vi "Get SysDef Configuration.vi"(8 "error in (no error)":errorcluster, 11 "Node Ptr":T27 format="%.0x") -> (0 "error out":errorcluster, 3 "Configuration":T1={"Name"="", "Description"="", "Protocol"="", "RS232 Config"={"Port"="COM1", "Baud Rate"=9600, "Data Bits"=8, "Parity"=enum."None", "Stop Bits"=10, "Flow Control"=0, "XON"=enum."DC1", "XOFF"=enum."DC3", "End Read on Termination Character"=TRUE, "End Write on Termination Character"=TRUE, "Termination Character"=10}, "MetaData Globals"=[], "Message Groups"=[], "GPIB Config"={"VISA Resource"="GPIB0::2::INSTR", "Enable Termination Character"=TRUE, "Termination Character"=10, "Timeout"=2000, "Append Write Termination Character"=FALSE}, "TCPIP Config"={"IP Address"="localhost", "Port"=0}, "Decimation"=0, "UDP Config"={"Local IP Address"="localhost", "Local Port"=8888, "Target IP Address"="localhost", "Target Port"=8888}} {"GPIB Config"."Termination Character" format="%.0x"; "RS232 Config"."Termination Character" format="%.0x"; "RS232 Config"."Flow Control" items=["None"=0, "XON/XOFF"=1, "RTS/CTS"=2, "DTR/DSR"=4]; "RS232 Config"."Stop Bits" items=["1.0"=10, "1.5"=15, "2.0"=20]; "RS232 Config"."Data Bits" min=5 max=8 step=1; "RS232 Config"."Baud Rate" items=["75"=75, "110"=110, "134"=134, "150"=150, "300"=300, "600"=600, "1200"=1200, "1800"=1800, "2400"=2400, "4800"=4800, "7200"=7200, "9600"=9600, "14400"=14400, "19200"=19200, "28800"=28800, "38400"=38400, "56000"=56000, "57600"=57600, "115200"=115200, "128000"=128000, "230400"=230400, "460800"=460800, "921600"=921600, "1843200"=1843200, "3000000"=3000000]})   [LabVIEW 2019, in "Instrument Addon System Explorer.lvlib"]
uses:
  Instrument Addon System Explorer.lvlib
  <vilib>/NI VeriStand/Custom Device API/Custom Device Item Ref.ctl
  Instrument Custom Device SysDef Configuration V1.0.1.ctl
  Shared/Types/RSXXX Port Settings.ctl
  MetaData Channel Configuration.ctl
  Shared/Types/MetaData Parameters.ctl
  Shared/Types/Protocol Data Type.ctl
  Shared/Types/Metadata Channel Type.ctl
  Shared/Types/Type Cast Type.ctl
  Shared/Types/Endian.ctl
  Types/Channel Properties.ctl
  Message Group Configuration.ctl
  Message Configuration.ctl
  Command Message Configuration.ctl
  Shared/Types/Command Parameters.ctl
  Shared/Types/Linked Channel Cluster.ctl
  Response Message Configuration.ctl
  Shared/Types/Response Parameters.ctl
  Shared/Types/Response Wait Type.ctl
  Data Channel Configuration.ctl
  Shared/Types/Data Parameters.ctl
  Shared/Types/Data Channel Type.ctl
  Shared/Types/Message Parameters.ctl
  Shared/Types/Message Generation Type.ctl
  Shared/Types/Trigger Parameters.ctl
  Shared/Types/VISA Settings.ctl
  Shared/Types/TCPIP Settings.ctl
  Shared/Types/UDP Settings.ctl
  Shared/Types/FG Control.ctl
  Shared/Constants.vi
  <vilib>/NI VeriStand/Custom Device API/Get Item Property (U32).vi
  <vilib>/NI VeriStand/Custom Device API/NI VeriStand - Set Item Property.vi
  <vilib>/NI VeriStand/Custom Device API/Set Item Property (U32).vi
  <vilib>/NI VeriStand/Custom Device API/Get Item Property (String).vi
  <vilib>/NI VeriStand/Custom Device API/Set Item Property (String).vi
  <vilib>/NI VeriStand/Custom Device API/Get Item Property (Boolean).vi
  <vilib>/NI VeriStand/Custom Device API/Set Item Property (Boolean).vi
  <vilib>/NI VeriStand/Custom Device Tools/Custom Device Utility Library/NI VeriStand - Search for Item by GUID.vi
  <vilib>/NI VeriStand/Custom Device API/Get Item Property (String Array).vi
  <vilib>/NI VeriStand/Custom Device API/Set Item Property (String Array).vi
  <vilib>/NI VeriStand/Custom Device API/NI VeriStand - Set Custom Device Channel Value Table.vi
  <vilib>/NI VeriStand/Custom Device Tools/Custom Device Utility Library/NI VeriStand - Search for All Items by GUID.vi
  <vilib>/NI VeriStand/Custom Device API/Get Item Property (Double).vi
  <vilib>/NI VeriStand/Custom Device API/Set Item Property (Double).vi
  <vilib>/NI VeriStand/Custom Device API/Custom Device API.lvlib
  Shared/Instrument Addon Shared.lvlib
  <vilib>/NI VeriStand/Custom Device Tools/Custom Device Utility Library/Custom Device Utility Library.lvlib
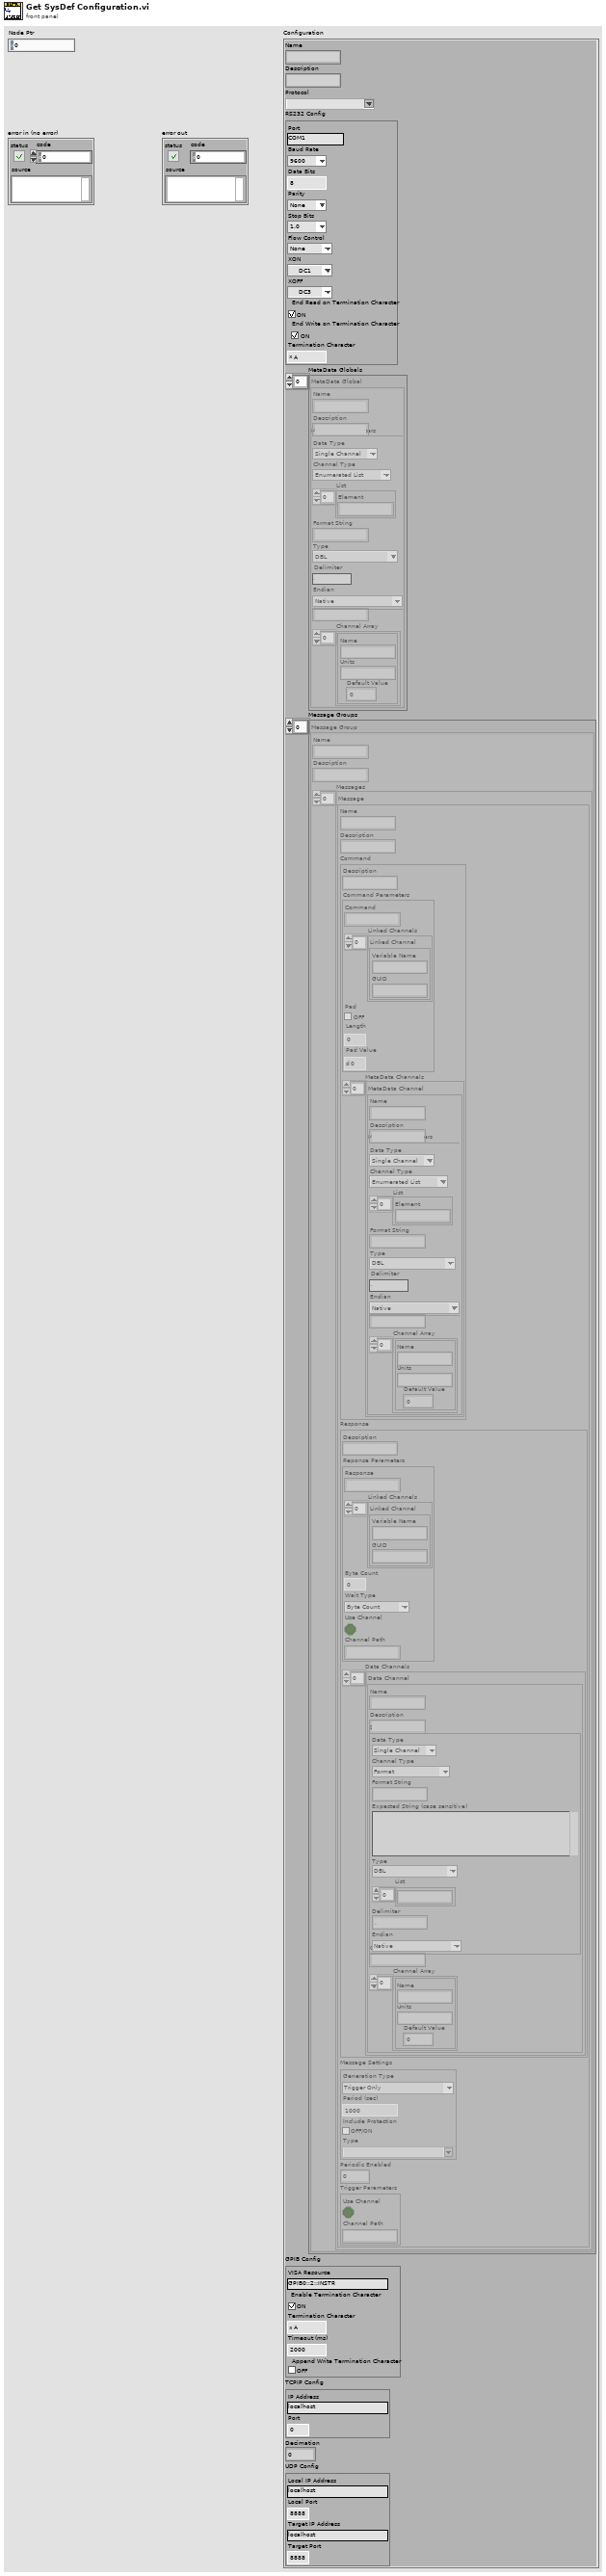
[diagram p1: front panel]
types:
  T1 = typedef "Instrument Addon System Explorer.lvlib/Instrument Custom Device SysDef Configuration V1.0.1.ctl" = cluster{"Name":string, "Description":string, "Protocol":string, "RS232 Config":T2, "MetaData Globals":T3[], "Message Groups":T10[], "GPIB Config":T24, "TCPIP Config":T25, "Decimation":u32, "UDP Config":T26}
  T2 = typedef "Instrument Addon Shared.lvlib/RSXXX Port Settings.ctl" = cluster{"Port":string, "Baud Rate":u32, "Data Bits":u16, "Parity":enum16{"None", "Odd", "Even", "Mark", "Space"}, "Stop Bits":u16, "Flow Control":u16, "XON":enum16{"NUL", "SOH", "STX", "ETX", "EOT", "ENQ", "ACK", "BEL", "BS", "HT", "LF", "VT", "FF", "CR", "SO", "SI", "DLE", "DC1", "DC2", "DC3", "DC4", "NAK", "SYN", "ETB", "CAN", "EM", "SUB", "ESC", "FS", "GS", "RS", "US", "SP", "!", "\"", "#", "$", "%", "&", "'", "(", ")", "*", "+", ",", "- (-)", ".", "/", "0", "1", "2", "3", "4", "5", "6", "7", "8", "9", ":", ";", "<", "=", ">", "?", "@", "A", "B", "C", "D", "E", "F", "G", "H", "I", "J", "K", "L", "M", "N", "O", "P", "Q", "R", "S", "T", "U", "V", "W", "X", "Y", "Z", "[", "\\", "]", "^", "_", "`", "a", "b", "c", "d", "e", "f", "g", "h", "i", "j", "k", "l", "m", "n", "o", "p", "q", "r", "s", "t", "u", "v", "w", "x", "y", "z", "{", "|", "}", "~"}, "XOFF":enum16{"NUL", "SOH", "STX", "ETX", "EOT", "ENQ", "ACK", "BEL", "BS", "HT", "LF", "VT", "FF", "CR", "SO", "SI", "DLE", "DC1", "DC2", "DC3", "DC4", "NAK", "SYN", "ETB", "CAN", "EM", "SUB", "ESC", "FS", "GS", "RS", "US", "SP", "!", "\"", "#", "$", "%", "&", "'", "(", ")", "*", "+", ",", "- (-)", ".", "/", "0", "1", "2", "3", "4", "5", "6", "7", "8", "9", ":", ";", "<", "=", ">", "?", "@", "A", "B", "C", "D", "E", "F", "G", "H", "I", "J", "K", "L", "M", "N", "O", "P", "Q", "R", "S", "T", "U", "V", "W", "X", "Y", "Z", "[", "\\", "]", "^", "_", "`", "a", "b", "c", "d", "e", "f", "g", "h", "i", "j", "k", "l", "m", "n", "o", "p", "q", "r", "s", "t", "u", "v", "w", "x", "y", "z", "{", "|", "}", "~"}, "End Read on Termination Character":bool, "End Write on Termination Character":bool, "Termination Character":u8}
  T3 = typedef "Instrument Addon System Explorer.lvlib/MetaData Channel Configuration.ctl" = cluster{"Name":string, "Description":string, "MetaData Parameters":T4, "Config GUID":string, "Channel Array":T9[]}
  T4 = typedef "Instrument Addon Shared.lvlib/MetaData Parameters.ctl" = cluster{"Data Type":T5, "Channel Type":T6, "List":string[], "Format String":string, "Type":T7, "Delimiter":string, "Endian":T8}
  T5 = typedef "Instrument Addon Shared.lvlib/Protocol Data Type.ctl" = enum16{"Single Channel", "Array"}
  T6 = typedef "Instrument Addon Shared.lvlib/Metadata Channel Type.ctl" = enum16{"Enumerated List", "Format", "Type Cast"}
  T7 = typedef "Instrument Addon Shared.lvlib/Type Cast Type.ctl" = enum16{"DBL", "SGL", "U64", "U32", "U16", "U8", "I64", "I32", "I16", "I8"}
  T8 = typedef "Instrument Addon Shared.lvlib/Endian.ctl" = enum16{"Native", "Little", "Big"}
  T9 = typedef "Instrument Addon System Explorer.lvlib/Channel Properties.ctl" = cluster{"Name":string, "Units":string, "Default Value":dbl}
  T10 = typedef "Instrument Addon System Explorer.lvlib/Message Group Configuration.ctl" = cluster{"Name":string, "Description":string, "Messages":T11[]}
  T11 = typedef "Instrument Addon System Explorer.lvlib/Message Configuration.ctl" = cluster{"Name":string, "Description":string, "Command":T12, "Response":T15, "Message Settings":T21, "Periodic Enabled":dbl, "Trigger Parameters":T23}
  T12 = typedef "Instrument Addon System Explorer.lvlib/Command Message Configuration.ctl" = cluster{"Description":string, "Command Parameters":T13, "MetaData Channels":T3[]}
  T13 = typedef "Instrument Addon Shared.lvlib/Command Parameters.ctl" = cluster{"Command":string, "Linked Channels":T14[], "Pad":bool, "Length":u32, "Pad Value":u8}
  T14 = typedef "Instrument Addon Shared.lvlib/Linked Channel Cluster.ctl" = cluster{"Variable Name":string, "GUID":string}
  T15 = typedef "Instrument Addon System Explorer.lvlib/Response Message Configuration.ctl" = cluster{"Description":string, "Reponse Parameters":T16, "Data Channels":T18[]}
  T16 = typedef "Instrument Addon Shared.lvlib/Response Parameters.ctl" = cluster{"Response":string, "Linked Channels":T14[], "Type Value":dbl, "Wait Type":T17, "Use Channel":bool, "Channel Path":string}
  T17 = typedef "Instrument Addon Shared.lvlib/Response Wait Type.ctl" = enum16{"Byte Count", "Wait sec"}
  T18 = typedef "Instrument Addon System Explorer.lvlib/Data Channel Configuration.ctl" = cluster{"Name":string, "Description":string, "Data Parameters":T19, "Config GUID":string, "Channel Array":T9[]}
  T19 = typedef "Instrument Addon Shared.lvlib/Data Parameters.ctl" = cluster{"Data Type":T5, "Channel Type":T20, "Format String":string, "Expected String":string, "Type":T7, "List":string[], "Delimiter":string, "Endian":T8}
  T20 = typedef "Instrument Addon Shared.lvlib/Data Channel Type.ctl" = enum16{"Format", "Comparison", "Type Cast", "Enumerated List"}
  T21 = typedef "Instrument Addon Shared.lvlib/Message Parameters.ctl" = cluster{"Generation Type":T22, "Period":dbl, "Include Protection":bool, "Type":string}
  T22 = typedef "Instrument Addon Shared.lvlib/Message Generation Type.ctl" = enum16{"Trigger Only", "Periodic & Trigger", "Value Change & Trigger"}
  T23 = typedef "Instrument Addon Shared.lvlib/Trigger Parameters.ctl" = cluster{"Use Channel":bool, "Channel Path":string}
  T24 = typedef "Instrument Addon Shared.lvlib/VISA Settings.ctl" = cluster{"VISA Resource":string, "Enable Termination Character":bool, "Termination Character":u8, "Timeout":u32, "Append Write Termination Character":bool}
  T25 = typedef "Instrument Addon Shared.lvlib/TCPIP Settings.ctl" = cluster{"IP Address":string, "Port":u16}
  T26 = typedef "Instrument Addon Shared.lvlib/UDP Settings.ctl" = cluster{"Local IP Address":string, "Local Port":u16, "Target IP Address":string, "Target Port":u16}
  T27 = typedef "Custom Device API.lvlib/Custom Device Item Ref.ctl" = u64
  T28 = typedef "Instrument Addon Shared.lvlib/FG Control.ctl" = enum16{"Get", "Set"}
  T29 = typedef "Custom Device API.lvlib/Custom Device Item Info.ctl" = cluster{"Name":string, "Is Channel":bool, "GUID":string, "Is Waveform":bool}
  T30 = typedef "Custom Device API.lvlib/Custom Device Channel.ctl" = cluster{"Type":T31, "Units":string, "Default Value":dbl, "Faultable":bool, "Scalable":bool}
  T31 = typedef "Custom Device API.lvlib/Custom Device Channel Type.ctl" = enum16{"Input", "Output"}
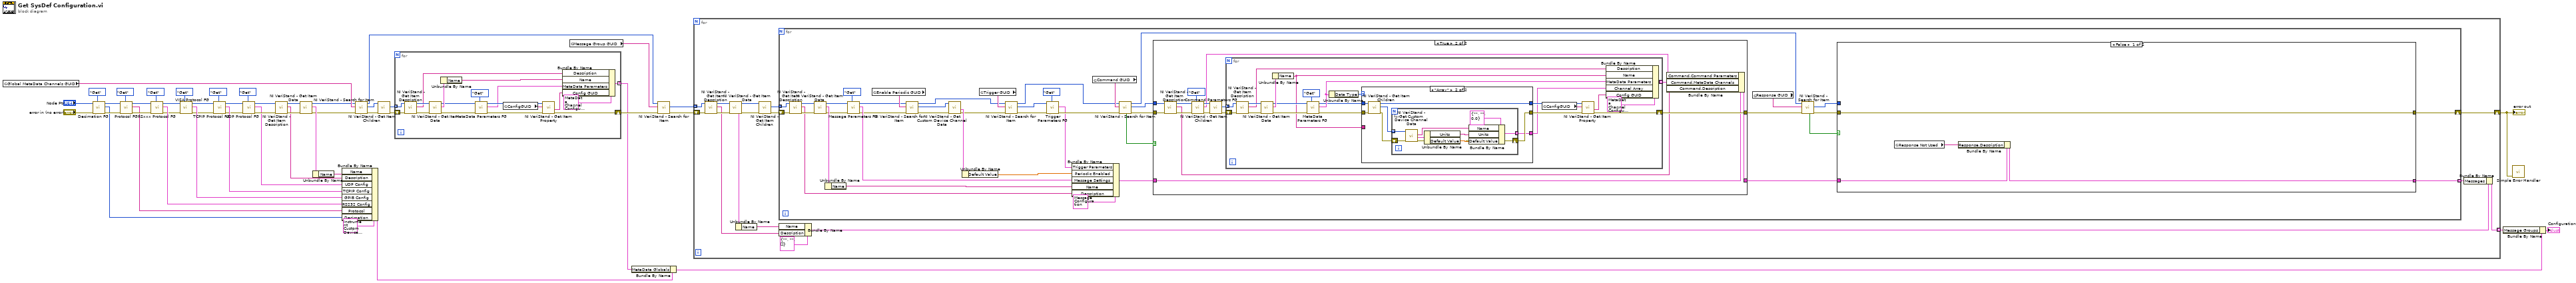
[diagram p0: block diagram]
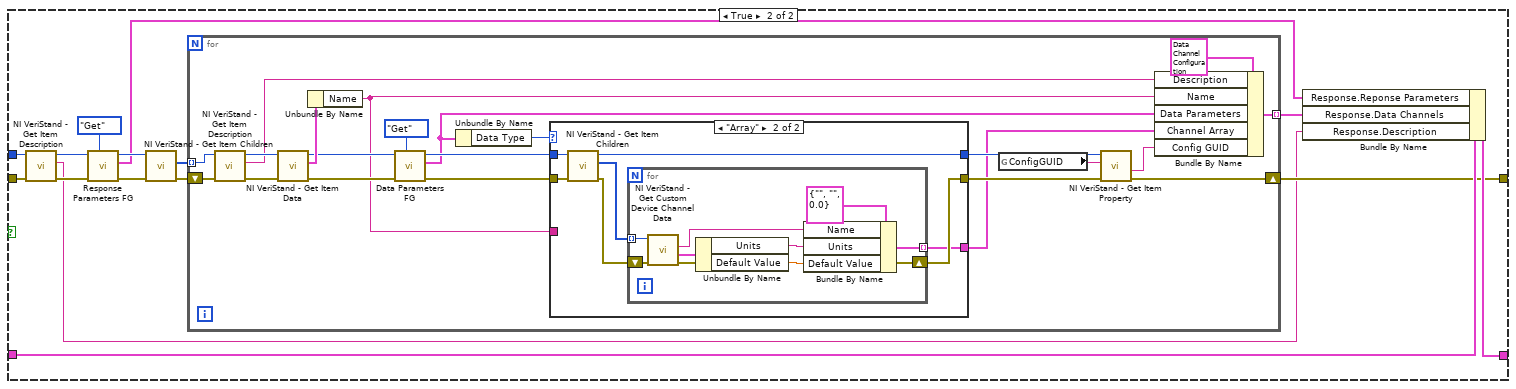
[diagram p2: hidden frame]
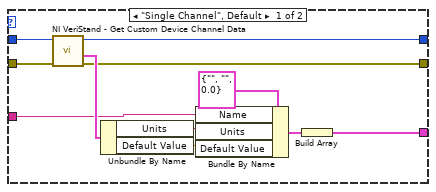
[diagram p3: hidden frame]
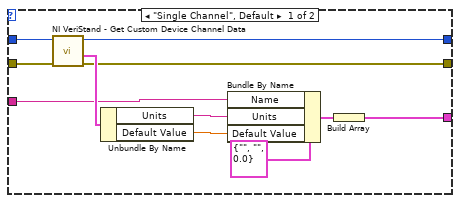
[diagram p5: hidden frame]
diagram:
  n1 = global read "Constants.vi" "Global MetaData Channels GUID"() -> (w46:string)
  n2 = call "Decimation FG.vi"("Action"=FG_Control."Get", "error in (no error)"="error in (no error)", "Device Item Ref in"="Node Ptr") -> ("error out"=w10:errorcluster, "Decimation out"=w7:u32, "Item Ref out"=w8:T27)  [unwired: 6 in]
  n3 = call "Protocol FG.vi"("Action"=FG_Control."Get", "error in (no error)"=w10, "Device Item Ref in"=w8) -> ("error out"=w43:errorcluster, "Protocol out"=w27:string, "Item Ref out"=w48:T27)  [unwired: 6 in]
  n4 = call "RSxxx Protocol FG.vi"("Action"=FG_Control."Get", "error in (no error)"=w43, "Device Item Ref in"=w48) -> ("error out"=w21:errorcluster, "Serial Config"=w25:T2, "Item Ref out"=w20:T27)  [unwired: 6 in]
  n5 = call "VISA Protocol FG.vi"("Action"=FG_Control."Get", "error in (no error)"=w21, "Device Item Ref in"=w20) -> ("error out"=w16:errorcluster, "VISA Config"=w19:T24, "Item Ref out"=w15:T27)  [unwired: 6 in]
  n6 = call "TCPIP Protocol FG.vi"("Action"=FG_Control."Get", "error in (no error)"=w16, "Device Item Ref in"=w15) -> ("error out"=w6:errorcluster, "TCP/IP Config"=w13:T25, "Item Ref out"=w4:T27)  [unwired: 6 in]
  n7 = call "UDP Protocol FG.vi"("Action"=FG_Control."Get", "error in (no error)"=w6, "Device Item Ref in"=w4) -> ("error out"=w5:errorcluster, "UDP Config"=w1:T26, "Item Ref out"=w3:T27)  [unwired: 6 in]
  n8 = call <vilib>:"NI VeriStand - Get Item Description.vi"("error in (no error)"=w5, "Item Ref in"=w3) -> ("error out"=w44:errorcluster, "Description"=w26:string, "Item Ref out"=w42:T27)  [unwired: 7 out]
  n9 = call <vilib>:"NI VeriStand - Get Item Data.vi"("error in (no error)"=w44, "Item Ref in"=w42) -> ("error out"=w40:errorcluster, "Item Info"=w50:T29, "Item Ref out"=w41:T27)  [unwired: 7 out]
  n10 = Unbundle By Name(w50) -> ("Name"=w24:string)
  n11 = Bundle By Name(cluster=T1 {"Name"="", "Description"="", "Protocol"="", "RS232 Config"={"Port"="", "Baud Rate"=0, "Data Bits"=0, "Parity"=enum."None", "Stop Bits"=0, "Flow Control"=0, "XON"=enum."NUL", "XOFF"=enum."NUL", "End Read on Termination Character"=FALSE, "End Write on Termination Character"=FALSE, "Termination Character"=0}, "MetaData Globals"=[], "Message Groups"=[], "GPIB Config"={"VISA Resource"="", "Enable Termination Character"=FALSE, "Termination Character"=0, "Timeout"=0, "Append Write Termination Character"=FALSE}, "TCPIP Config"={"IP Address"="", "Port"=0}, "Decimation"=0, "UDP Config"={"Local IP Address"="", "Local Port"=0, "Target IP Address"="", "Target Port"=0}}, "Name"=w24, "Description"=w26, "UDP Config"=w1, "TCPIP Config"=w13, "GPIB Config"=w19, "RS232 Config"=w25, "Protocol"=w27, "Decimation"=w7) -> (w22:T1)
  n12 = call-poly <vilib>:"NI VeriStand - Search for Item.vi"("error in"=w40, "Item GUID"=w46, "Section Ref in"=w41) -> ("error out"=w38:errorcluster, "Item Ref"=w45:T27, "Section Ref out"=w34:T27)  [unwired: 5 in, 1 out]
  n13 = call <vilib>:"NI VeriStand - Get Item Children.vi"("error in (no error)"=w38, "Item Ref in"=w45) -> ("error out"=w37:errorcluster, "Child Refs"=w39:T27[])  [unwired: 6 in, 2 out]
  n14 = for {
    tunnel: w39 -> [w65] mode=indexing
    shift-right: [w57] -> w35
    shift-left: w37 -> [w64]
    tunnel: [w51] -> w31 mode=indexing
    n15 = call <vilib>:"NI VeriStand - Get Item Description.vi"("error in (no error)"=w64, "Item Ref in"=w65) -> ("error out"=w67:errorcluster, "Description"=w52:string, "Item Ref out"=w68:T27)  [unwired: 7 out]
    n16 = call <vilib>:"NI VeriStand - Get Item Data.vi"("error in (no error)"=w67, "Item Ref in"=w68) -> ("error out"=w59:errorcluster, "Item Info"=w66:T29, "Item Ref out"=w58:T27)  [unwired: 7 out]
    n17 = Unbundle By Name(w66) -> ("Name"=w53:string)
    n18 = call "MetaData Parameters FG.vi"("Action"=FG_Control."Get", "error in (no error)"=w59, "Item Ref in"=w58) -> ("error out"=w61:errorcluster, "MetaData Parameters"=w54:T4, "Item Ref out"=w60:T27)  [unwired: 6 in]
    n19 = global read "Constants.vi" "ConfigGUID"() -> (w62:string)
    n20 = call-poly <vilib>:"NI VeriStand - Get Item Property.vi"("error in (no error)"=w61, "Property Name"=w62, "Item Ref in"=w60) -> ("error out"=w57:errorcluster, "Value"=w55:string)  [unwired: 5 in, 2 out]
    n21 = Bundle By Name(cluster=T3 {"Name"="", "Description"="", "MetaData Parameters"={"Data Type"=enum."Single Channel", "Channel Type"=enum."Enumerated List", "List"=[], "Format String"="", "Type"=enum."DBL", "Delimiter"="", "Endian"=enum."Native"}, "Config GUID"="", "Channel Array"=[]}, "Description"=w52, "Name"=w53, "MetaData Parameters"=w54, "Config GUID"=w55) -> (w51:T3)
  }
  n22 = global read "Constants.vi" "Message Group GUID"() -> (w36:string)
  n23 = Bundle By Name(cluster=w22, "MetaData Globals"=w31) -> (w30:T1)
  n24 = call-poly <vilib>:"NI VeriStand - Search for Item.vi"("error in"=w35, "Item GUID"=w36, "Section Ref in"=w34) -> ("error out"=w33:errorcluster, "Item Refs"=w32:T27[])  [unwired: 5 in, 2 out]
  n25 = for {
    tunnel: w32 -> [w80] mode=indexing
    tunnel: [w70] -> w29 mode=indexing
    shift-right: [w69] -> w17
    shift-left: w33 -> [w81]
    n26 = call <vilib>:"NI VeriStand - Get Item Description.vi"("error in (no error)"=w81, "Item Ref in"=w80) -> ("error out"=w83:errorcluster, "Description"=w73:string, "Item Ref out"=w82:T27)  [unwired: 7 out]
    n27 = call <vilib>:"NI VeriStand - Get Item Data.vi"("error in (no error)"=w83, "Item Ref in"=w82) -> ("error out"=w78:errorcluster, "Item Info"=w84:T29, "Item Ref out"=w79:T27)  [unwired: 7 out]
    n28 = Unbundle By Name(w84) -> ("Name"=w74:string)
    n29 = call <vilib>:"NI VeriStand - Get Item Children.vi"("error in (no error)"=w78, "Item Ref in"=w79) -> ("error out"=w77:errorcluster, "Child Refs"=w76:T27[])  [unwired: 6 in, 2 out]
    n30 = for {
      tunnel: w76 -> [w121] mode=indexing
      tunnel: [w112] -> w72 mode=indexing
      shift-right: [w111] -> w69
      shift-left: w77 -> [w122]
      n31 = call <vilib>:"NI VeriStand - Get Item Description.vi"("error in (no error)"=w122, "Item Ref in"=w121) -> ("error out"=w124:errorcluster, "Description"=w115:string, "Item Ref out"=w125:T27)  [unwired: 7 out]
      n32 = call <vilib>:"NI VeriStand - Get Item Data.vi"("error in (no error)"=w124, "Item Ref in"=w125) -> ("error out"=w103:errorcluster, "Item Info"=w123:T29, "Item Ref out"=w102:T27)  [unwired: 7 out]
      n33 = Unbundle By Name(w123) -> ("Name"=w116:string)
      n34 = call "Message Parameters FG.vi"("Action"=FG_Control."Get", "error in (no error)"=w103, "Item Ref in"=w102) -> ("error out"=w99:errorcluster, "Message Settings out"=w100:T21, "Item Ref out"=w98:T27)  [unwired: 6 in]
      n35 = global read "Constants.vi" "Enable Periodic GUID"() -> (w104:string)
      n36 = call-poly <vilib>:"NI VeriStand - Search for Item.vi"("error in"=w99, "Item GUID"=w104, "Section Ref in"=w98) -> ("error out"=w97:errorcluster, "Item Ref"=w95:T27, "Section Ref out"=w91:T27)  [unwired: 5 in, 1 out]
      n37 = call <vilib>:"NI VeriStand - Get Custom Device Channel Data.vi"("error in (no error)"=w97, "Channel Ref in"=w95) -> ("error out"=w92:errorcluster, "Channel"=w94:T30)  [unwired: 4 in, 4 out]
      n38 = Unbundle By Name(w94) -> ("Default Value"=w96:dbl)
      n39 = global read "Constants.vi" "Trigger GUID"() -> (w93:string)
      n40 = call-poly <vilib>:"NI VeriStand - Search for Item.vi"("error in"=w92, "Item GUID"=w93, "Section Ref in"=w91) -> ("error out"=w90:errorcluster, "Item Ref"=w88:T27, "Section Ref out"=w87:T27)  [unwired: 5 in, 1 out]
      n41 = call "Trigger Parameters FG.vi"("Action"=FG_Control."Get", "error in (no error)"=w90, "Item Ref in"=w88) -> ("error out"=w89:errorcluster, "Trigger Parameters"=w86:T23)  [unwired: 6 in, 1 out]
      n42 = Bundle By Name(cluster=T11 {"Name"="", "Description"="", "Command"={"Description"="", "Command Parameters"={"Command"="", "Linked Channels"=[], "Pad"=FALSE, "Length"=0, "Pad Value"=0}, "MetaData Channels"=[]}, "Response"={"Description"="", "Reponse Parameters"={"Response"="", "Linked Channels"=[], "Type Value"=0.0, "Wait Type"=enum."Byte Count", "Use Channel"=FALSE, "Channel Path"=""}, "Data Channels"=[]}, "Message Settings"={"Generation Type"=enum."Trigger Only", "Period"=0.0, "Include Protection"=FALSE, "Type"=""}, "Periodic Enabled"=0.0, "Trigger Parameters"={"Use Channel"=FALSE, "Channel Path"=""}}, "Trigger Parameters"=w86, "Periodic Enabled"=w96, "Message Settings"=w100, "Name"=w116, "Description"=w115) -> (w114:T11)
      n43 = global read "Constants.vi" "Command GUID"() -> (w126:string)
      n44 = call-poly <vilib>:"NI VeriStand - Search for Item.vi"("error in"=w89, "Item GUID"=w126, "Section Ref in"=w87) -> ("error out"=w109:errorcluster, "Item Ref"=w110:T27, "Section Ref out"=w118:T27, "Found"=w106:bool)  [unwired: 5 in]
      n45 = case shown="True" w106 {
        tunnel: [w195 w206] -> w119
        tunnel: w114 -> [w196 w203]
        tunnel: [w196 w202] -> w113
        tunnel: w110 -> [_ w201]
        tunnel: w109 -> [w195 w200]
        frame False {
        }
        frame True {
          n46 = call <vilib>:"NI VeriStand - Get Item Description.vi"("error in (no error)"=w200, "Item Ref in"=w201) -> ("error out"=w199:errorcluster, "Description"=w197:string, "Item Ref out"=w198:T27)  [unwired: 7 out]
          n47 = call "Command Parameters FG.vi"("Action"=FG_Control."Get", "error in (no error)"=w199, "Item Ref in"=w198) -> ("error out"=w210:errorcluster, "Command Parameters"=w205:T13, "Item Ref out"=w207:T27)  [unwired: 6 in]
          n48 = call <vilib>:"NI VeriStand - Get Item Children.vi"("error in (no error)"=w210, "Item Ref in"=w207) -> ("error out"=w209:errorcluster, "Child Refs"=w208:T27[])  [unwired: 6 in, 2 out]
          n49 = for {
            tunnel: w208 -> [w230] mode=indexing
            shift-right: [w224] -> w206
            shift-left: w209 -> [w229]
            tunnel: [w220] -> w204 mode=indexing
            n50 = call <vilib>:"NI VeriStand - Get Item Description.vi"("error in (no error)"=w229, "Item Ref in"=w230) -> ("error out"=w232:errorcluster, "Description"=w221:string, "Item Ref out"=w233:T27)  [unwired: 7 out]
            n51 = call <vilib>:"NI VeriStand - Get Item Data.vi"("error in (no error)"=w232, "Item Ref in"=w233) -> ("error out"=w226:errorcluster, "Item Info"=w231:T29, "Item Ref out"=w225:T27)  [unwired: 7 out]
            n52 = Unbundle By Name(w231) -> ("Name"=w213:string)
            n53 = call "MetaData Parameters FG.vi"("Action"=FG_Control."Get", "error in (no error)"=w226, "Item Ref in"=w225) -> ("error out"=w215:errorcluster, "MetaData Parameters"=w219:T4, "Item Ref out"=w217:T27)  [unwired: 6 in]
            n54 = Unbundle By Name(w219) -> ("Data Type"=w218:T5)
            n55 = case shown="\"Array\"" w218 {
              tunnel: w217 -> [w241 w251]
              tunnel: [w240 w250] -> w216
              tunnel: w215 -> [w243 w249]
              tunnel: [w242 w246] -> w214
              tunnel: [w235 w245] -> w212
              tunnel: w213 -> [w237 _]
              frame "Single Channel", Default {
                n56 = call <vilib>:"NI VeriStand - Get Custom Device Channel Data.vi"("error in (no error)"=w243, "Channel Ref in"=w241) -> ("error out"=w242:errorcluster, "Channel"=w244:T30, "Channel Ref out"=w240:T27)  [unwired: 4 in, 3 out]
                n57 = Unbundle By Name(w244) -> ("Units"=w238:string, "Default Value"=w239:dbl)
                n58 = Bundle By Name(cluster=T9 {"Name"="", "Units"="", "Default Value"=0.0}, "Name"=w237, "Units"=w238, "Default Value"=w239) -> (w236:T9)
                n59 = Build Array(w236) -> (w235:T9[])
              }
              frame "Array" {
                n60 = call <vilib>:"NI VeriStand - Get Item Children.vi"("error in (no error)"=w249, "Item Ref in"=w251) -> ("error out"=w247:errorcluster, "Child Refs"=w248:T27[], "Item Ref out"=w250:T27)  [unwired: 6 in, 1 out]
                n61 = for {
                  tunnel: w248 -> [w260] mode=indexing
                  tunnel: [w255] -> w245 mode=indexing
                  shift-right: [w253] -> w246
                  shift-left: w247 -> [w254]
                  n62 = call <vilib>:"NI VeriStand - Get Custom Device Channel Data.vi"("error in (no error)"=w254, "Channel Ref in"=w260) -> ("error out"=w253:errorcluster, "Channel"=w259:T30, "Channel Name"=w258:string)  [unwired: 4 in, 3 out]
                  n63 = Unbundle By Name(w259) -> ("Units"=w257:string, "Default Value"=w256:dbl)
                  n64 = Bundle By Name(cluster=T9 {"Name"="", "Units"="", "Default Value"=0.0}, "Name"=w258, "Units"=w257, "Default Value"=w256) -> (w255:T9)
                }
              }
            }
            n65 = global read "Constants.vi" "ConfigGUID"() -> (w227:string)
            n66 = call-poly <vilib>:"NI VeriStand - Get Item Property.vi"("error in (no error)"=w214, "Property Name"=w227, "Item Ref in"=w216) -> ("error out"=w224:errorcluster, "Value"=w222:string)  [unwired: 5 in, 2 out]
            n67 = Bundle By Name(cluster=T3 {"Name"="", "Description"="", "MetaData Parameters"={"Data Type"=enum."Single Channel", "Channel Type"=enum."Enumerated List", "List"=[], "Format String"="", "Type"=enum."DBL", "Delimiter"="", "Endian"=enum."Native"}, "Config GUID"="", "Channel Array"=[]}, "Description"=w221, "Name"=w213, "MetaData Parameters"=w219, "Channel Array"=w212, "Config GUID"=w222) -> (w220:T3)
          }
          n68 = Bundle By Name(cluster=w203, "Command.Command Parameters"=w205, "Command.MetaData Channels"=w204, "Command.Description"=w197) -> (w202:T11)
        }
      }
      n69 = global read "Constants.vi" "Response GUID"() -> (w120:string)
      n70 = call-poly <vilib>:"NI VeriStand - Search for Item.vi"("error in"=w119, "Item GUID"=w120, "Section Ref in"=w118) -> ("error out"=w108:errorcluster, "Item Ref"=w107:T27, "Found"=w105:bool)  [unwired: 5 in, 1 out]
      n71 = case shown="False" w105 {
        tunnel: w113 -> [w129 w138]
        tunnel: [w128 w137] -> w112
        tunnel: [w130 w136] -> w111
        tunnel: w108 -> [w130 w135]
        tunnel: w107 -> [_ w133]
        frame False {
          n72 = global read "Constants.vi" "Response Not Used"() -> (w127:string)
          n73 = Bundle By Name(cluster=w129, "Response.Description"=w127) -> (w128:T11)
        }
        frame True {
          n74 = call <vilib>:"NI VeriStand - Get Item Description.vi"("error in (no error)"=w135, "Item Ref in"=w133) -> ("error out"=w134:errorcluster, "Description"=w131:string, "Item Ref out"=w132:T27)  [unwired: 7 out]
          n75 = call "Response Parameters FG.vi"("Action"=FG_Control."Get", "error in (no error)"=w134, "Item Ref in"=w132) -> ("error out"=w142:errorcluster, "Reponse Parameters"=w139:T16, "Item Ref out"=w141:T27)  [unwired: 6 in]
          n76 = call <vilib>:"NI VeriStand - Get Item Children.vi"("error in (no error)"=w142, "Item Ref in"=w141) -> ("error out"=w144:errorcluster, "Child Refs"=w145:T27[])  [unwired: 6 in, 2 out]
          n77 = for {
            tunnel: w145 -> [w164] mode=indexing
            shift-right: [w161] -> w136
            shift-left: w144 -> [w163]
            tunnel: [w154] -> w140 mode=indexing
            n78 = call <vilib>:"NI VeriStand - Get Item Description.vi"("error in (no error)"=w163, "Item Ref in"=w164) -> ("error out"=w166:errorcluster, "Description"=w156:string, "Item Ref out"=w167:T27)  [unwired: 7 out]
            n79 = call <vilib>:"NI VeriStand - Get Item Data.vi"("error in (no error)"=w166, "Item Ref in"=w167) -> ("error out"=w159:errorcluster, "Item Info"=w165:T29, "Item Ref out"=w158:T27)  [unwired: 7 out]
            n80 = Unbundle By Name(w165) -> ("Name"=w146:string)
            n81 = call "Data Parameters FG.vi"("Action"=FG_Control."Get", "error in (no error)"=w159, "Item Ref in"=w158) -> ("error out"=w153:errorcluster, "Data Parameters"=w149:T19, "Item Ref out"=w151:T27)  [unwired: 6 in]
            n82 = Unbundle By Name(w149) -> ("Data Type"=w148:T5)
            n83 = case shown="\"Array\"" w148 {
              tunnel: w151 -> [w175 w185]
              tunnel: [w174 w184] -> w150
              tunnel: w153 -> [w177 w183]
              tunnel: [w176 w180] -> w152
              tunnel: [w169 w179] -> w147
              tunnel: w146 -> [w171 _]
              frame "Single Channel", Default {
                n84 = call <vilib>:"NI VeriStand - Get Custom Device Channel Data.vi"("error in (no error)"=w177, "Channel Ref in"=w175) -> ("error out"=w176:errorcluster, "Channel"=w178:T30, "Channel Ref out"=w174:T27)  [unwired: 4 in, 3 out]
                n85 = Unbundle By Name(w178) -> ("Units"=w172:string, "Default Value"=w173:dbl)
                n86 = Bundle By Name(cluster=T9 {"Name"="", "Units"="", "Default Value"=0.0}, "Name"=w171, "Units"=w172, "Default Value"=w173) -> (w170:T9)
                n87 = Build Array(w170) -> (w169:T9[])
              }
              frame "Array" {
                n88 = call <vilib>:"NI VeriStand - Get Item Children.vi"("error in (no error)"=w183, "Item Ref in"=w185) -> ("error out"=w181:errorcluster, "Child Refs"=w182:T27[], "Item Ref out"=w184:T27)  [unwired: 6 in, 1 out]
                n89 = for {
                  tunnel: w182 -> [w194] mode=indexing
                  tunnel: [w189] -> w179 mode=indexing
                  shift-right: [w187] -> w180
                  shift-left: w181 -> [w188]
                  n90 = call <vilib>:"NI VeriStand - Get Custom Device Channel Data.vi"("error in (no error)"=w188, "Channel Ref in"=w194) -> ("error out"=w187:errorcluster, "Channel"=w193:T30, "Channel Name"=w192:string)  [unwired: 4 in, 3 out]
                  n91 = Unbundle By Name(w193) -> ("Units"=w191:string, "Default Value"=w190:dbl)
                  n92 = Bundle By Name(cluster=T9 {"Name"="", "Units"="", "Default Value"=0.0}, "Name"=w192, "Units"=w191, "Default Value"=w190) -> (w189:T9)
                }
              }
            }
            n93 = global read "Constants.vi" "ConfigGUID"() -> (w162:string)
            n94 = call-poly <vilib>:"NI VeriStand - Get Item Property.vi"("error in (no error)"=w152, "Property Name"=w162, "Item Ref in"=w150) -> ("error out"=w161:errorcluster, "Value"=w155:string)  [unwired: 5 in, 2 out]
            n95 = Bundle By Name(cluster=T18 {"Name"="", "Description"="", "Data Parameters"={"Data Type"=enum."Single Channel", "Channel Type"=enum."Format", "Format String"="", "Expected String"="", "Type"=enum."DBL", "List"=[], "Delimiter"="", "Endian"=enum."Native"}, "Config GUID"="", "Channel Array"=[]}, "Description"=w156, "Name"=w146, "Data Parameters"=w149, "Channel Array"=w147, "Config GUID"=w155) -> (w154:T18)
          }
          n96 = Bundle By Name(cluster=w138, "Response.Reponse Parameters"=w139, "Response.Data Channels"=w140, "Response.Description"=w131) -> (w137:T11)
        }
      }
    }
    n97 = Bundle By Name(cluster=T10 {"Name"="", "Description"="", "Messages"=[]}, "Name"=w74, "Description"=w73) -> (w71:T10)
    n98 = Bundle By Name(cluster=w71, "Messages"=w72) -> (w70:T10)
  }
  "error out" <- w17
  n99 = Bundle By Name(cluster=w30, "Message Groups"=w29) -> (→"Configuration":T1)
  n100 = call <vilib>:"Simple Error Handler.vi"("error in (no error)"=w17) -> ()  [unwired: 4 in, 5 out]
